vi "initialise.vi"(8 "error in (no error)":errorcluster, 11 "GenericPlugin in":refnum<class "LightSourceMH110124MaiTai.lvclass">) -> (0 "error out":errorcluster, 3 "GenericPlugin out":refnum<class "LightSourceMH110124MaiTai.lvclass">)   [LabVIEW 2010, in "LightSourceMH110124MaiTai.lvclass"]
doc: "The dynamic dispatch-version of this VI initalises the plug-in object by allocating and initalising any dynamic resources need."
uses:
  LightSourceMH110124MaiTai.lvclass
  LightSourceScaffold/LightSourceScaffold/LightSourceScaffold.lvclass
  LightSourceMH110124MaiTai.lvclass/LightSourceMH110124MaiTai.ctl
  <vilib>/Instr/_visa.llb/VISA Configure Serial Port (Instr).vi
  class_data.vi
  common/classes/ErrorController/ErrorController/class_data.vi
  common/classes/ErrorController/ErrorController/ErrorController.lvclass
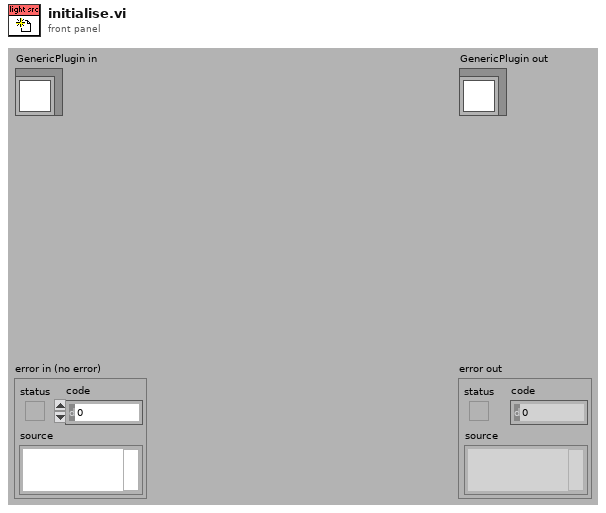
[diagram p1: front panel]
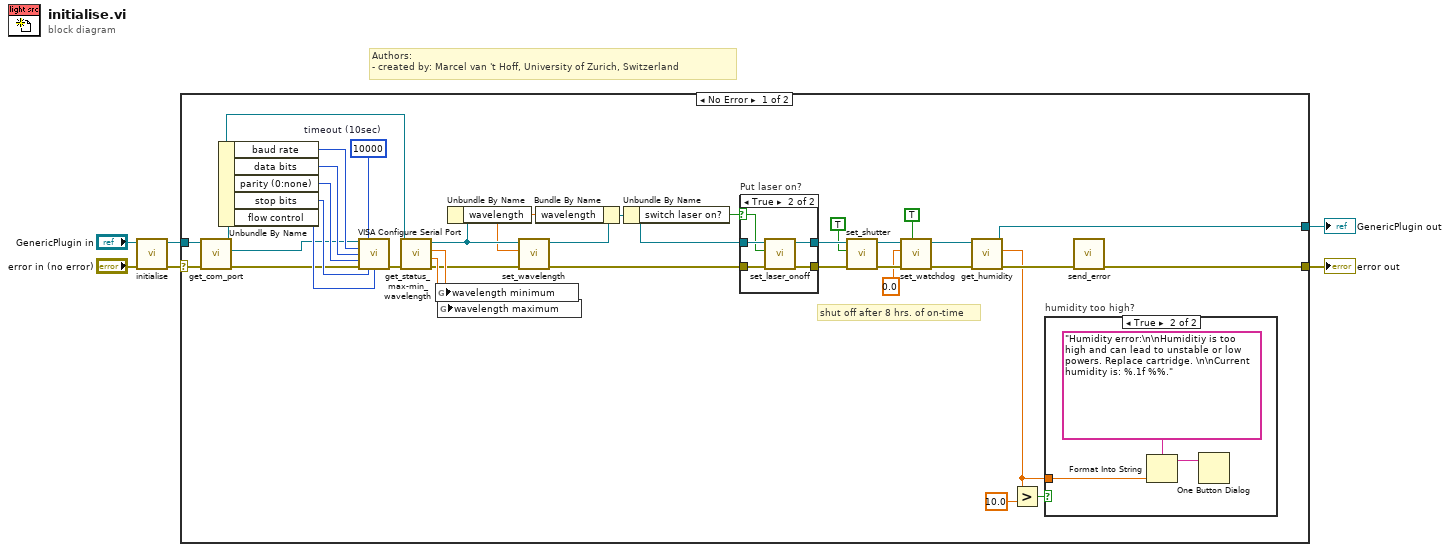
[diagram p0: block diagram]
diagram:
  # "Authors: \n- created by: Marcel van 't Hoff, University of Zurich, Switzerland"
  n1 = call-parent "initialise.vi"("error in (no error)"="error in (no error)", "GenericPlugin in"="GenericPlugin in") -> ("error out"=w1:errorcluster, "GenericPlugin out"=w3:refnum<class "LightSourceMH110124MaiTai.lvclass">)  [unwired: 8 in]
  n2 = case shown="No Error" w1 {
    selector: w1 -> [w30 w54]
    tunnel: [w26 w54] -> w6
    tunnel: [w12 w53] -> w5
    tunnel: w3 -> [w31 w53]
    frame No Error {
      w37 = u32 10000  # timeout (10sec)
      # "shut off after 8 hrs. of on-time"
      n3 = call-dynamic "get_com_port.vi"("error in (no error)"=w30, "LightSourceMH110124MaiTai in"=w31) -> ("error out"=w29:errorcluster, "comm port"=w28:refnum<visa-resource-name>, "LightSourceMH110124MaiTai out"=w27:refnum<class "LightSourceMH110124MaiTai.lvclass">)  [unwired: 7 in]
      n4 = Unbundle By Name(w27) -> ("baud rate"=w38:u32, "data bits"=w39:u16, "parity (0:none)"=w40:enum16{"None", "Odd", "Even", "Mark", "Space"}, "stop bits"=w41:u16, "flow control"=w42:u16)
      n5 = call-poly "VISA Configure Serial Port"("VISA resource name"=w28, "timeout (10sec)"=w37, "baud rate (9600)"=w38, "data bits (8)"=w39, "parity (0:none)"=w40, "error in (no error)"=w29, "stop bits (10: 1 bit)"=w41, "flow control (0:none)"=w42) -> ("error out"=w36:errorcluster)  [unwired: 1 in, 6 out]
      n6 = call-dynamic "get_status_max-min_wavelength.vi"("error in (no error)"=w36, "LightSourceMH110124MaiTai in"=w27) -> ("error out"=w22:errorcluster, "maximal wavelength out"=w24:dbl[unit], "minimal wavelength out"=w25:dbl[unit], "LightSourceMH110124MaiTai out"=w23:refnum<class "LightSourceMH110124MaiTai.lvclass">)  [unwired: 6 in]
      n7 = global write "class_data.vi" "wavelength minimum"(w25) -> ()
      n8 = global write "class_data.vi" "wavelength maximum"(w24) -> ()
      n9 = Unbundle By Name(w23) -> ("wavelength"=w19:dbl[unit])
      n10 = call-dynamic "set_wavelength.vi"("error in (no error)"=w22, "wavelength in"=w19, "LightSourceMH110124MaiTai in"=w23) -> ("error out"=w21:errorcluster, "LightSourceMH110124MaiTai out"=w20:refnum<class "LightSourceMH110124MaiTai.lvclass">)  [unwired: 7 in]
      n11 = Bundle By Name(cluster=w20, "wavelength"=w19) -> (w18:refnum<class "LightSourceMH110124MaiTai.lvclass">)
      n12 = Unbundle By Name(w18) -> ("switch laser on?"=w35:bool)
      n13 = case "Put laser on?" shown="True" w35 {
        selector: w35 -> [_ w50]
        tunnel: w21 -> [w46 w52]
        tunnel: w18 -> [w47 w51]
        tunnel: [w46 w49] -> w33
        tunnel: [w47 w48] -> w34
        frame False {
        }
        frame True {
          n14 = call-dynamic "set_laser_onoff.vi"("error in (no error)"=w52, "on?"=w50, "LightSourceMH110124MaiTai in"=w51) -> ("error out"=w49:errorcluster, "LightSourceMH110124MaiTai out"=w48:refnum<class "LightSourceMH110124MaiTai.lvclass">)  [unwired: 7 in]
        }
      }
      n15 = call-dynamic "set_shutter.vi"("error in (no error)"=w33, "shutter open?"=TRUE, "LightSourceMH110124MaiTai in"=w34) -> ("error out"=w16:errorcluster, "LightSourceMH110124MaiTai out"=w17:refnum<class "LightSourceMH110124MaiTai.lvclass">)  [unwired: 6 in, 1 out]
      n16 = call-dynamic "set_watchdog.vi"("set watchdog on/off (F)"=TRUE, "error in (no error)"=w16, "set timer"=dbl[unit] 0.0, "LightSourceMH110124MaiTai in"=w17) -> ("error out"=w11:errorcluster, "LightSourceMH110124MaiTai out"=w13:refnum<class "LightSourceMH110124MaiTai.lvclass">)  [unwired: 6 in]
      n17 = call-dynamic "get_humidity.vi"("error in (no error)"=w11, "LightSourceMH110124MaiTai in"=w13) -> ("error out"=w10:errorcluster, "humidity"=w7:dbl, "LightSourceMH110124MaiTai out"=w12:refnum<class "LightSourceMH110124MaiTai.lvclass">)  [unwired: 7 in]
      n18 = Greater?(x=w7, y=10.0) -> (0:w8:bool)
      n19 = case "humidity too high?" shown="True" w8 {
        tunnel: w7 -> [_ w45]
        frame False {
        }
        frame True {
          n20 = Format Into String(format string="Humidity error:\n\nHumiditiy is too high and can lead to unstable or low powers. Replace cartridge. \n\nCurrent humidity is: %.1f %%.", w45) -> (resulting string=w43:string)  [unwired: 2 in, 1 out]
          n21 = One Button Dialog(message=w43) -> ()  [unwired: 1 in, 1 out]
        }
      }
      n22 = call "send_error.vi"("error in (no error)"=w10) -> ("error out"=w26:errorcluster)  [unwired: 10 in]
    }
    frame Error {
    }
  }
  "error out" <- w6
  "GenericPlugin out" <- w5
